vi "Write CAN FIFO.vi"(4 "T_Out":u64, 6 "T0":u64, 8 "error in (no error)":errorcluster, 9 "Timeout (ms)":i32, 10 "Data":T1[](array[typedef]) {"Tags" format="%.0x"; "payload" format="%x"; "identifier" format="%x"}, 11 "CIFTag in":refnum<class "CIF_NIChn_FifoCAN.lvclass">) -> (0 "error out":errorcluster, 1 "timed out?":bool, 3 "CIFTag out":refnum<class "CIF_NIChn_FifoCAN.lvclass">)   [LabVIEW 2021, in "CIF_NIChn_FifoCAN.lvclass"]
uses:
  CIF_NIChn_FifoCAN.lvclass
  D:/dev/CIF-LVCore/src/Channels/CIFChannels/CIFChannels.lvclass
  D:/dev/CIF-LVCore/src/Channels/CIF_NIChn/NIChn/CIF_NIChn.lvclass
  ChannelCommon/typedef/Datatype CAN.ctl
  CIFChannels/CIFChannels.lvclass/CIFChannels.ctl
  CIF_NIChn_FifoCAN.lvclass/CIF_NIChn_FifoCAN.ctl
  ChannelCommon/CIFFIFO/CIFfifo.lvclass/CIFfifo.ctl
  NIChn/CIF_NIChn.lvclass/CIF_NIChn.ctl
  ChannelCommon/CIFFIFO/Accessors/Read Length.vi
  <vilib>/CIFChannels/SubVIs/Get dll Path.vi
  ChannelCommon/CIFFIFO/Utilities/Update Header.vi
  ChannelCommon/CIFFIFO/Flatten/CAN Flatten.vi
  ChannelCommon/CIFFIFO/Accessors/Write T0.vi
  ChannelCommon/CIFFIFO/Accessors/Write T_Out.vi
  CIFChannels/Accessors/Read ClockID.vi
  ChannelCommon/Utilities/Flatten Header.vi
  ChannelCommon/CIFFIFO/Flatten/CAN Flatten.vi/be899675-9489-4ae7-9bdb-bbc908cd9623.vi
  ChannelCommon/CIFFIFO/Flatten/CAN Flatten.vi/fa4e04b0-1c28-4039-87e0-9391600efeb5.vi
  ChannelCommon/CIFFIFO/Flatten/CAN Flatten.vi/24dfac9c-4f7b-471b-adb6-3e40fb284e05.vi
  ChannelCommon/CIFFIFO/Accessors/Write Payload Length.vi
  ChannelCommon/CIFFIFO/Accessors/Read Header.vi
  CIFCore/Common/Utilities/Add Error.vi
  ChannelCommon/CIFFIFO/Flatten/CAN Flatten.vi/be899675-9489-4ae7-9bdb-bbc908cd9623.vi/c28b0ead-42ad-4072-80a2-aca7f2bd7ce3.vi
  ChannelCommon/CIFFIFO/Flatten/CAN Flatten.vi/fa4e04b0-1c28-4039-87e0-9391600efeb5.vi/c28b0ead-42ad-4072-80a2-aca7f2bd7ce3.vi
  ChannelCommon/CIFFIFO/Flatten/CAN Flatten.vi/24dfac9c-4f7b-471b-adb6-3e40fb284e05.vi/c28b0ead-42ad-4072-80a2-aca7f2bd7ce3.vi
  CIFCore/Common/Utilities/Append Error Location.vi
  ChannelCommon/Utilities/Update Time.vi
  NIChn/CIF_NIChn.lvclass
  <vilib>/CIFChannels/CIFChannelCore.lvlib
  ChannelCommon/CIFFIFO/CIFfifo.lvclass
  ChannelCommon/ChannelCommon.lvlib
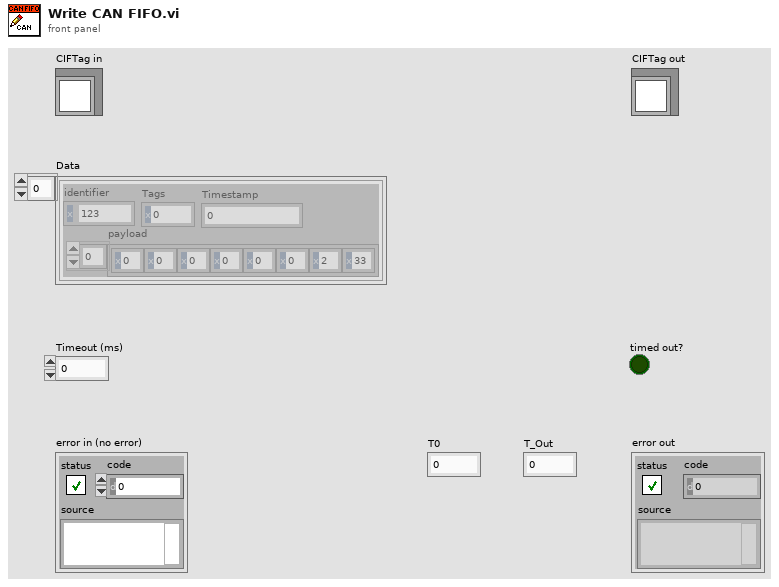
[diagram p1: front panel]
types:
  T1 = typedef "ChannelCommon.lvlib/Datatype CAN.ctl" = cluster{"payload":u8[], "identifier":u32, "Tags":u8, "Timestamp":u64}
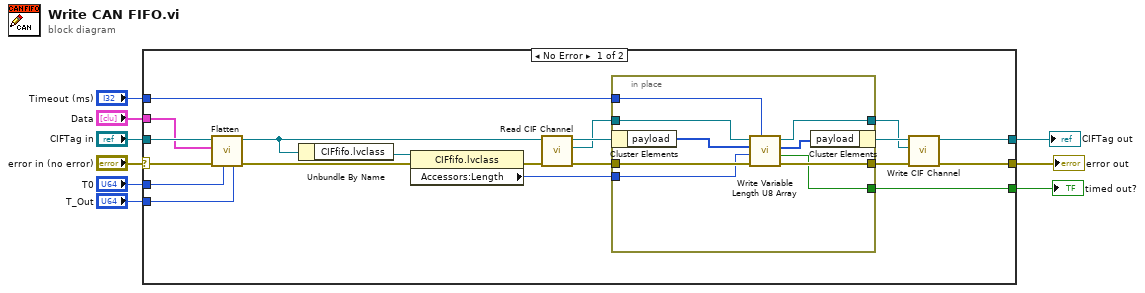
[diagram p0: block diagram]
diagram:
  n1 = case shown="No Error" "error in (no error)" {
    selector: "error in (no error)" -> [w14 w40]
    tunnel: [w20 w40] -> w8
    tunnel: [w25 w39] -> w6
    tunnel: "CIFTag in" -> [w17 w39]
    tunnel: [w29 _] -> w5
    tunnel: "Timeout (ms)" -> [w21 _]
    tunnel: "T_Out" -> [w12 _]
    tunnel: "T0" -> [w13 _]
    tunnel: "Data" -> [w10 _]
    frame No Error {
      n2 = call "Flatten.vi"("T_Out"=w12, "T0"=w13, "error in (no error)"=w14, "Data in"=w10, "CIFTag in"=w17) -> ("error out"=w15:errorcluster, "CIFTag out"=w16:refnum<class "CIF_NIChn_FifoCAN.lvclass">)  [unwired: 5 in]
      n3 = Unbundle By Name(w16) -> ("CIFfifo.lvclass"=w19:refnum<class "CIFfifo.lvclass">)
      n4 = property class="CIFfifo.lvclass"(reference=w19, error in=w15) -> (error out=w18:errorcluster, "Accessors:Length"=w11:u64)  [unwired: 1 out]
      n5 = call "Read CIF Channel.vi"("error in (no error)"=w18, "CIFTag in"=w16) -> ("error out"=w27:errorcluster, "CIF Channel"=w23:refnum<k21>, "CIFTag out"=w28:refnum<class "CIF_NIChn_FifoCAN.lvclass">)  [unwired: 7 in]
      n6 = in-place {
        in-place-border: w27 -> [w38]
        in-place-border: [w37] -> w24
        in-place-border: [w36] -> w29
        in-place-border: w23 -> [w35]
        in-place-border: [w34] -> w22
        in-place-border: w21 -> [w33]
        in-place-border: w11 -> [w31]
        n7 = in-place-cluster #1(w28) -> ("payload"=w32:u8[])
        n8 = call <vilib>:"Write Variable Length U8 Array.vi"("Timeout (ms)"=w33, "error in"=w38, "numElements"=w31, "U8 Array in"=w32, "CIF Channel in"=w35) -> ("error out"=w37:errorcluster, "Timed out?"=w36:bool, "U8 Array out"=w30:u8[], "CIF Channel out"=w34:refnum<k21>)  [unwired: 3 in]
        n9 = in-place-cluster #1("payload"=w30) -> (w26:refnum<class "CIF_NIChn_FifoCAN.lvclass">)
      }
      n10 = call "Write CIF Channel.vi"("error in (no error)"=w24, "CIF Channel"=w22, "CIFTag in"=w26) -> ("error out"=w20:errorcluster, "CIFTag out"=w25:refnum<class "CIF_NIChn_FifoCAN.lvclass">)  [unwired: 7 in]
    }
    frame Error {
    }
  }
  "error out" <- w8
  "CIFTag out" <- w6
  "timed out?" <- w5
